vi "DAQ_Close.vi"(8 "error in (no error)":errorcluster, 11 "DAQ Prams":T1={"task in"="", "Num Pts"=0, "timeout"=0.0, "FIFO"=0, "Double Bounce"=1.0, "Sensitivity (V/X)"=[]} {"Double Bounce" format="%#.2g"}) -> (0 "error out":errorcluster)   [LabVIEW 2022 SP3]
uses:
  <vilib>/Utility/error.llb/DialogType.ctl
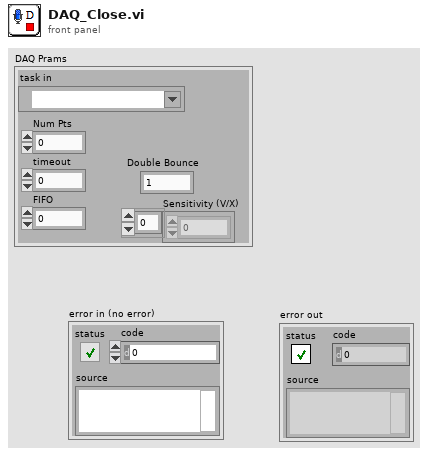
[diagram p1: front panel]
types:
  T1 = cluster{"task in":refnum<k21>, "Num Pts":i32, "timeout":dbl, "FIFO":i32, "Double Bounce":dbl, "Sensitivity (V/X)":dbl[]}
  T2 = typedef "DialogType.ctl" = u16
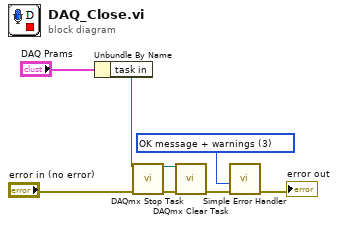
[diagram p0: block diagram]
diagram:
  w4 = T2 3 items=["no dialog", "OK message", "continue or stop message", "OK message + warnings", "continue/stop + warnings"] ("type of dialog (OK msg:1)")
  n1 = Unbundle By Name("DAQ Prams") -> ("task in"=w2:refnum<k21>)
  n2 = call <vilib>:"DAQmx Stop Task.vi"("task/channels in"=w2, "error in"="error in (no error)") -> ("task out"=w6:refnum<k21>, "error out"=w5:errorcluster)  [unwired: 12 in]
  n3 = call <vilib>:"DAQmx Clear Task.vi"("task in"=w6, "error in"=w5) -> ("error out"=w7:errorcluster)  [unwired: 13 in]
  n4 = call <vilib>:"Simple Error Handler.vi"("type of dialog (OK msg:1)"=w4, "error in (no error)"=w7) -> ("error out"=→"error out":errorcluster)  [unwired: 3 in, 4 out]
